vi "Add All Channels.vi"(8 "error in (no error)":errorcluster, 10 "Number of CPU Cores in":u64, 11 "Item Ref in":T1 format="%.0x") -> (0 "error out":errorcluster, 3 "Item Ref out":T1 format="%.0x")   [LabVIEW 2027, in "System Monitor System Explorer.lvlib"]
uses:
  System Monitor System Explorer.lvlib
  <vilib>/NI VeriStand/Custom Device API/Custom Device Item Ref.ctl
  <vilib>/NI VeriStand/Custom Device API/Custom Device API.lvlib
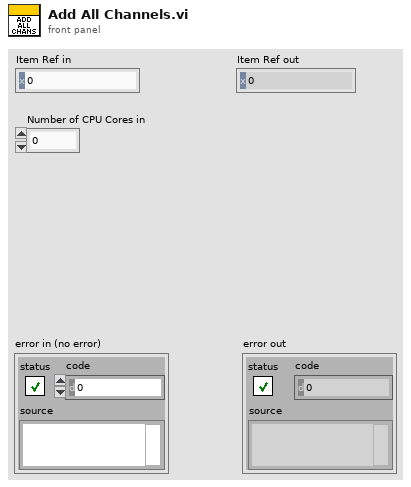
[diagram p1: front panel]
types:
  T1 = typedef "Custom Device API.lvlib/Custom Device Item Ref.ctl" = u64
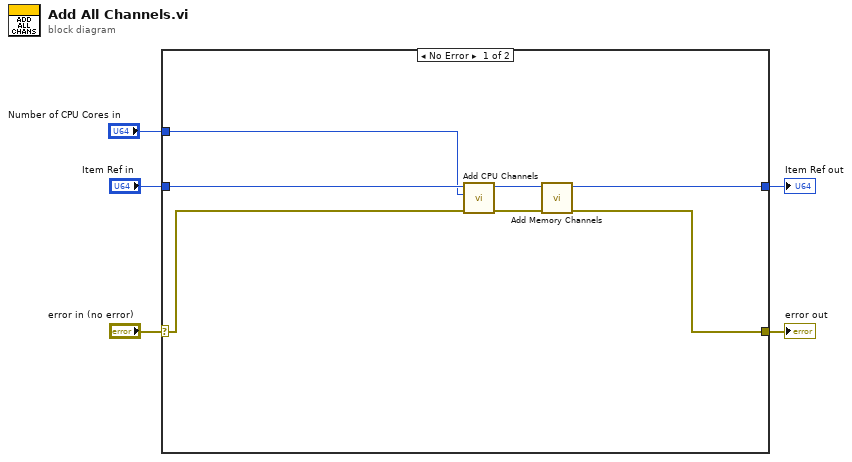
[diagram p0: block diagram]
diagram:
  n1 = case shown="No Error" "error in (no error)" {
    selector: "error in (no error)" -> [w6 w14]
    tunnel: [w9 w14] -> w5
    tunnel: [w8 w13] -> w3
    tunnel: "Item Ref in" -> [w11 w13]
    tunnel: "Number of CPU Cores in" -> [w7 _]
    frame No Error {
      n2 = call "Add CPU Channels.vi"("error in (no error)"=w6, "Number of CPU Cores in"=w7, "Item Ref in"=w11) -> ("error out"=w10:errorcluster, "Item Ref out"=w12:T1)  [unwired: 7 in]
      n3 = call "Add Memory Channels.vi"("error in (no error)"=w10, "Item Ref in"=w12) -> ("error out"=w9:errorcluster, "Item Ref out"=w8:T1)  [unwired: 8 in]
    }
    frame Error {
    }
  }
  "error out" <- w5
  "Item Ref out" <- w3
